vi "Validate Command Refnum.vi"(8 "error in (no error)":errorcluster, 11 "command refnum in":T1 format="%.0x") -> (0 "error out":errorcluster, 3 "command refnum out":T1 format="%.0x")   [LabVIEW 2020, in "Instrument Addon Scripting API.lvlib"]
uses:
  Instrument Addon Scripting API.lvlib
  <vilib>/NI VeriStand/Custom Device API/Custom Device Item Ref.ctl
  Shared Directory/Constants.vi
  Dependencies.llb/Instrument_Addon_Scripting_Dependencies_Advanced System Definition.lvlib
  Shared Directory/Instrument Addon Shared.lvlib
  <vilib>/NI VeriStand/Custom Device API/Custom Device API.lvlib
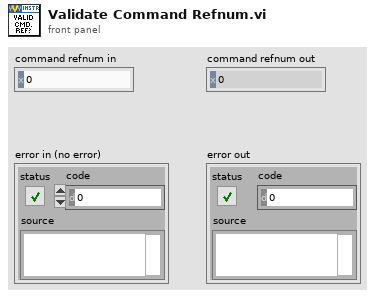
[diagram p1: front panel]
types:
  T1 = typedef "Custom Device API.lvlib/Custom Device Item Ref.ctl" = u64
  T2 = typedef "Instrument_Addon_Scripting_Dependencies_Advanced System Definition.lvlib/Instrument_Addon_Scripting_Dependencies_TreeItem.Info.ctl" = cluster{"Name":string, "Description":string, "GUID":string, "Is Channel":bool, "Channel":T3, "Is Waveform":bool, "Waveform":T5}
  T3 = typedef "Custom Device API.lvlib/Custom Device Channel.ctl" = cluster{"Type":T4, "Units":string, "Default Value":dbl, "Faultable":bool, "Scalable":bool}
  T4 = typedef "Custom Device API.lvlib/Custom Device Channel Type.ctl" = enum16{"Input", "Output"}
  T5 = typedef "Custom Device API.lvlib/Custom Device Waveform.ctl" = cluster{"Data Type":T6, "Units":string}
  T6 = typedef "Custom Device API.lvlib/Custom Device Waveform DataType.ctl" = enum16{"Double", "Complex Double"}
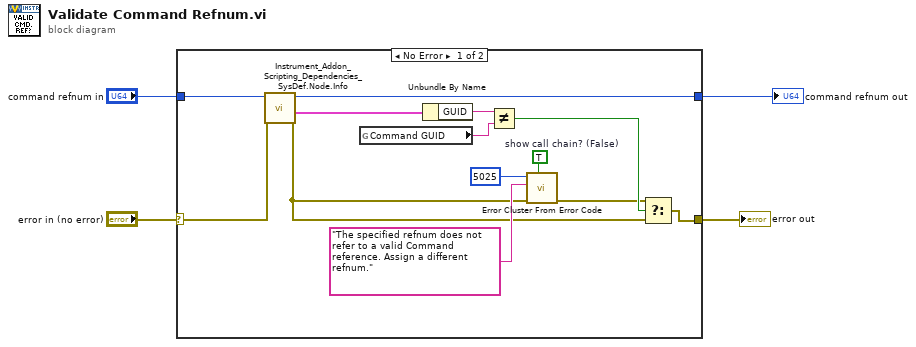
[diagram p0: block diagram]
diagram:
  n1 = case shown="No Error" "error in (no error)" {
    selector: "error in (no error)" -> [w11 w18]
    tunnel: [w15 w19] -> w1
    tunnel: "command refnum in" -> [w13 w19]
    tunnel: [w10 w18] -> w2
    frame No Error {
      w8 = TRUE  # show call chain? (False)
      n2 = call "Instrument_Addon_Scripting_Dependencies_SysDef.Node.Info.vi"("error in (no error)"=w11, "nodeID"=w13) -> ("error out"=w5:errorcluster, "Item Info"=w14:T2, "nodeID out"=w15:u64)  [unwired: 6 in, 1 out]
      n3 = global read "Constants.vi" "Command GUID"() -> (w17:string)
      n4 = Unbundle By Name(w14) -> ("GUID"=w16:string)
      n5 = Not Equal?(x=w16, y=w17) -> (x != y?=w12:bool)
      n6 = call <vilib>:"Error Cluster From Error Code.vi"("show call chain? (False)"=w8, "error in (no error)"=w5, "error message (\"\")"="The specified refnum does not refer to a valid Command reference. Assign a different refnum." ("error message (\"\")"), "error code (0)"=5025) -> ("error out"=w9:errorcluster)  [unwired: 5 in]
      n7 = Select(t=w9, s=w12, f=w5) -> (s? t:f=w10:errorcluster)
    }
    frame Error {
    }
  }
  "error out" <- w2
  "command refnum out" <- w1
